vi "Get Value by Array (JSON).vi"(8 "error in (no error)":errorcluster, 10 "Keys":string[](array[string]), 11 "JSON Value in":refnum<class "JSON Value.lvclass">) -> (0 "error out":errorcluster, 2 "JSON Value out":refnum<class "JSON Value.lvclass">)   [LabVIEW 2016, in "JSON Value.lvclass"]
uses:
  JSON Value.lvclass
  subVIs/Errors.ctl
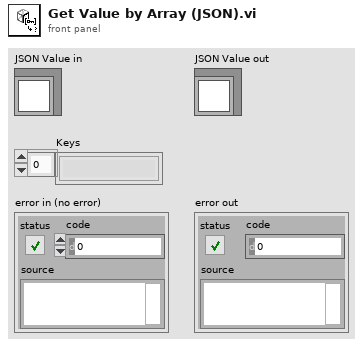
[diagram p1: front panel]
types:
  T1 = typedef "JSON Value.lvclass/Errors.ctl" = enum16{"No key", "Key path type", "Array OOB", "Type Mismatch", "Invalid Token"}
  T2 = typedef "JSON Value.lvclass/JSON Types.ctl" = enum16{"String", "Numeric", "Boolean", "NULL", "Object", "Array"}
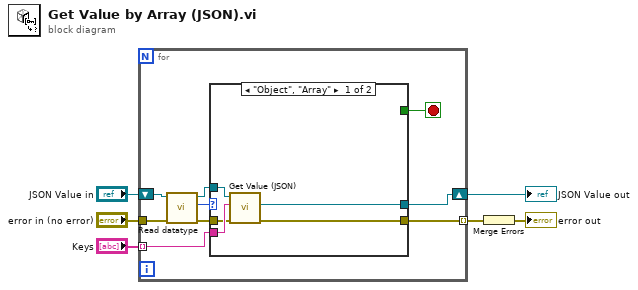
[diagram p0: block diagram]
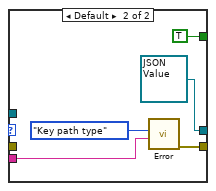
[diagram p2: hidden frame]
diagram:
  n1 = for {
    tunnel: "Keys" -> [w15] mode=indexing
    shift-right: [w14] -> w5
    shift-left: "JSON Value in" -> [w11]
    tunnel: "error in (no error)" -> [w8]
    tunnel: [w13] -> w2 mode=indexing
    stop <- w12 stop-if-true
    n2 = call "Read datatype.vi"("error in (no error)"=w8, "JSON Datatype in"=w11) -> ("error out"=w9:errorcluster, "datatype"=w7:T2, "JSON Datatype out"=w10:refnum<class "JSON Value.lvclass">)  [unwired: 7 in]
    n3 = case shown="\"Object\", \"Array\"" w7 {
      tunnel: w15 -> [w20 w22]
      tunnel: [w19 refnum<class "JSON Value.lvclass"> refnum ("JSON out")] -> w14
      tunnel: w10 -> [w16 _]
      tunnel: [w17 w24] -> w13
      tunnel: w9 -> [w18 _]
      tunnel: [_ TRUE] -> w12
      frame "Object", "Array" {
        n4 = call "Get Value (JSON).vi"("error in (no error)"=w18, "key"=w20, "JSON Value in"=w16) -> ("error out"=w17:errorcluster, "JSON Value out"=w19:refnum<class "JSON Value.lvclass">)  [unwired: 7 in]
      }
      frame Default {
        n5 = call "Error.vi"("Data"=w22, 9:Errors."Key path type") -> ("error out"=w24:errorcluster)  [unwired: 8 in]
      }
    }
  }
  "JSON Value out" <- w5
  n6 = Merge Errors(w2) -> (→"error out":errorcluster)
